vi "After Launch Init.vi"(8 "error in (no error)":errorcluster, 11 "CS++GoBangClient in":refnum<class "CS++GoBangClient.lvclass">) -> (0 "error out":errorcluster, 3 "CS++GoBangClient out":refnum<class "CS++GoBangClient.lvclass">)   [LabVIEW 2013, in "GoBang.lvlib" / "CS++GoBangClient.lvclass"]
doc: "Use <b>Pre Launch init.vi</b> method only for sanity checks that are supposed to prevent the actor from launching if they fail. Use <B>this</B> method instead to initialize unique resources that must be released during the <b>Stop Core.vi</b> method. A corresponding high priority message will become dispatched before the <B>Actor Framework.lvlib:Actor.lvclass.Actor Core.vi</b> is called.\n\n<b>Derived classed should call the parent methode first</b> and their own initialization code after.\n\nRefer also to the ongoing discussion at https://decibel.ni.com/content/message/57394#57394."
uses:
  CS++GoBangClient.lvclass
  Core/Actors/CS++BaseActor/CS++BaseActor.lvclass
  CS++GoBangClient.lvclass/CS++GoBangClient.ctl
  Core/Classes/CS++ProcessVariables/PVConnection/PVConnection.lvclass/PVConnection.ctl
  Core/Classes/CS++ProcessVariables/PVConnection/PVConnection.lvclass
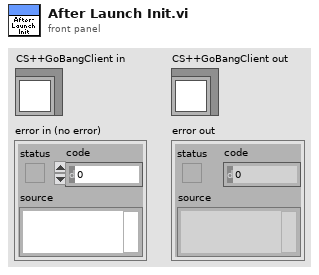
[diagram p1: front panel]
types:
  T1 = cluster{"Write Access":enum8{"Allowed", "Required", "None"}, "Read Access":enum8{"Allowed", "Required", "None"}}
  T2 = cluster{"JoinGame":refnum<class "PVConnection.lvclass">, "UpdateBoard":refnum<class "PVConnection.lvclass">}
  T3 = cluster{"[0]":refnum<class "PVConnection.lvclass">, "[1]":refnum<class "PVConnection.lvclass">}
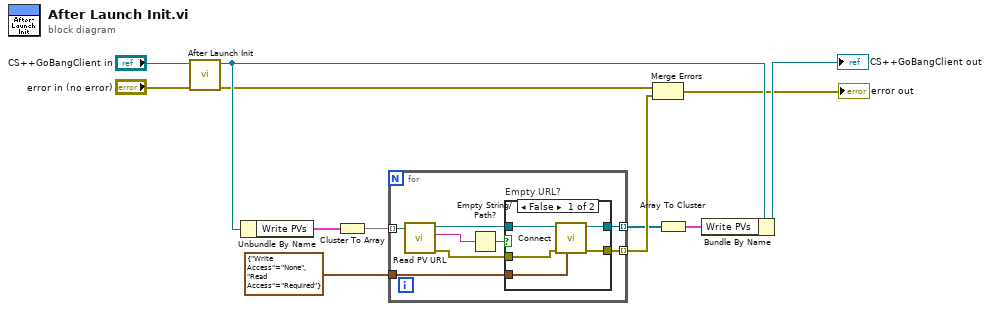
[diagram p0: block diagram]
diagram:
  n1 = call-parent "After Launch Init.vi"("error in (no error)"="error in (no error)", "CS++BaseActor in"="CS++GoBangClient in") -> ("error out"=w1:errorcluster, "CS++BaseActor out"=w4:refnum<class "CS++GoBangClient.lvclass">)  [unwired: 8 in]
  n2 = Unbundle By Name(w4) -> ("Write PVs"=w6:T2)
  n3 = Cluster To Array(cluster=w6) -> (array=w8:refnum<class "PVConnection.lvclass">[])
  n4 = for {
    tunnel: w8 -> [w16] mode=indexing
    tunnel: T1 {"Write Access"=enum."None", "Read Access"=enum."Required"} ("Access") -> [w20]
    tunnel: [w19] -> w9 mode=indexing
    tunnel: [w17] -> w10 mode=indexing
    n5 = call "Read PV URL.vi"("PVConnection in"=w16) -> ("error out"=w13:errorcluster, "PV URL"=w14:string, "PVConnection out"=w15:refnum<class "PVConnection.lvclass">)  [unwired: 8 in]
    n6 = Empty String/Path?(string/path=w14) -> (empty?=w18:bool)
    n7 = case "Empty URL?" shown="False" w18 {
      tunnel: w15 -> [w25 w26]
      tunnel: w20 -> [w23 _]
      tunnel: [w24 w26] -> w19
      tunnel: [w22 _] -> w17
      tunnel: w13 -> [w21 _]
      frame False {
        n8 = call-dynamic "Connect.vi"("Access"=w23, "error in (no error)"=w21, "PVConnection in"=w25) -> ("error out"=w22:errorcluster, "PVConnection out"=w24:refnum<class "PVConnection.lvclass">)  [unwired: 7 in]
      }
      frame True {
      }
    }
  }
  n9 = Merge Errors(w1, w10) -> (→"error out":errorcluster)
  n10 = Array To Cluster(array=w9) -> (cluster=w7:T3)
  n11 = Bundle By Name(cluster=w4, "Write PVs"=w7) -> (→"CS++GoBangClient out":refnum<class "CS++GoBangClient.lvclass">)
